vi "Periodic Tasks.vi"(8 "error in":errorcluster) -> ()   [LabVIEW 2017]
doc: "This VI runs in parallel to other tasks. It can contain as many user-defined periodic loops as you need. These can carry out PID or other sorts of timed response."
uses:
  <vilib>/Rock Robotics/WPI/Utilities/WPI_GetSetVariantRefNum.vi
  <vilib>/Rock Robotics/Network Tables/NT Write Numeric Array.vi
  <vilib>/Rock Robotics/Network Tables/NT Write Number.vi
  <vilib>/Rock Robotics/WPI/ThirdParty/Phoenix-LabVIEW/Motor Controller/Get/CTRE_Phoenix_MotorController_GetQuadratureData.vi
  <vilib>/Rock Robotics/WPI/ThirdParty/Phoenix-LabVIEW/Motor Controller/Get/CTRE_Phoenix_MotorController_GetOutputCurrent_Enhanced.vi
  <vilib>/Rock Robotics/WPI/ThirdParty/Phoenix-LabVIEW/Motor Controller/Get/CTRE_Phoenix_MotorController_GetVoltage.vi
  <vilib>/Rock Robotics/WPI/ThirdParty/Phoenix-LabVIEW/Motor Controller/Get/CTRE_Phoenix_MotorController_GetTemperature.vi
  <vilib>/Rock Robotics/Network Tables/NT Write Variant.vi
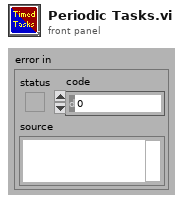
[diagram p1: front panel]
types:
  T1 = typedef "WPI_JoystickDevRef.ctl" = cluster{"Device":T2}
  T2 = typedef "WPI_JoystickDeviceEnum.ctl" = enum16{"USB 0", "USB 1", "USB 2", "USB 3", "USB 4", "USB 5"}
  T3 = typedef "WPI_AccelerometerDevRef.ctl" = cluster{"DevStatus":errorcluster, "Scaling":T4, "Analog Channels":T5, "I2C Bus":T7, "SPI Bus":T8, "Accel Range":T9, "ADXL Axes":T10, "Handle":i32, "Device Address":u8, "Accel Type":enum16{"Analog", "ADXL345 I2C", "ADXL345 SPI", "Internal", "ADXL362 SPI"}}
  T4 = typedef "WPI_AccelerometerScaling.ctl" = cluster{"Gain (VoltsPerG)":dbl, "Center Voltage":dbl}
  T5 = typedef "WPI_AccelerometerAnalogChannels.ctl" = cluster{"X-Axis":T6, "Y-Axis":T6, "Z-Axis":T6}
  T6 = typedef "FPGA_AIChannel.ctl" = enum8{"AI 0", "AI 1", "AI 2", "AI 3", "AI MXP 0", "AI MXP 1", "AI MXP 2", "AI MXP 3", "Invalid"}
  T7 = typedef "i2c_bus.ctl" = enum16{"I2C On-Board", "I2C MXP", "Invalid"}
  T8 = typedef "spi_bus.ctl" = enum16{"SPI On-Board, CS0", "SPI On-Board, CS1", "SPI On-Board, CS2", "SPI On-Board, CS3", "SPI MXP", "Invalid"}
  T9 = typedef "ADXL345 Range.ctl" = u8
  T10 = typedef "WPI_AccelerometerADXL345 Axes.ctl" = cluster{"X-Axis":bool, "Y-Axis":bool, "Z-Axis":bool}
  T11 = cluster{"X-Axis":dbl, "Y-Axis":dbl, "Z-Axis":dbl}
  T12 = typedef "WPI_GyroDevRef.ctl" = cluster{"DevStatus":errorcluster, "Analog Channel":T6, "Gain (VoltsPerDegree/Second)":dbl, "Gyro Type":enum16{"Analog", "XRS450"}, "Handle":i32, "SPI Bus":T8, "Device Found":bool, "Sample Rate":dbl, "Calibrate On Open":bool, "Offset":dbl}
  T13 = typedef "WPI_MotorControlDeviceRef.ctl" = cluster{"DeviceStatus":errorcluster, "Type":T14, "PWM":cluster{"PWM Channel":T15, "DeadBand":T16}, "CAN":cluster{"Device Number":u8, "SetOutput VI Ref":variant, "GetOutput VI Ref":variant, "Enable VI Ref":variant, "Disable VI Ref":variant, "Data":variant}, "Invert":bool, "DIO PWM":cluster{"PWM \"Enable\" Channel":T15, "DIOChannel":T17, "PWM Rate":dbl}}
  T14 = typedef "WPI_MotorControlType.ctl" = enum16{"PWM", "CAN", "DIO PWM"}
  T15 = typedef "FPGA_DIOPWMChannel.ctl" = enum8{"PWM 0", "PWM 1", "PWM 2", "PWM 3", "PWM 4", "PWM 5", "PWM 6", "PWM 7", "PWM 8", "PWM 9", "PWM MXP 0", "PWM MXP 1", "PWM MXP 2", "PWM MXP 3", "PWM MXP 4", "PWM MXP 5", "PWM MXP 6", "PWM MXP 7", "PWM MXP 8", "PWM MXP 9", "Invalid"}
  T16 = typedef "WPI_PWMDeadband.ctl" = cluster{"Name":string, "maxPositivePwm":i32, "minPositivePwm":i32, "centerPwm":i32, "maxNegativePwm":i32, "minNegativePwm":i32, "angularRange":u16}
  T17 = typedef "FPGA_DIOChannel.ctl" = enum8{"DIO 0", "DIO 1", "DIO 2", "DIO 3", "DIO 4", "DIO 5", "DIO 6", "DIO 7", "DIO 8", "DIO 9", "DIO MXP 0", "DIO MXP 1", "DIO MXP 2", "DIO MXP 3", "DIO MXP 4", "DIO MXP 5", "DIO MXP 6", "DIO MXP 7", "DIO MXP 8", "DIO MXP 9", "DIO MXP 10", "DIO MXP 11", "DIO MXP 12", "DIO MXP 13", "DIO MXP 14", "DIO MXP 15", "SPI Port CS1", "SPI Port CS2", "SPI Port CS3", "SPI Port MISO", "SPI Port MOSI", "Invalid"}
  T18 = cluster{"Temperature (C)":dbl, "Percent Output":dbl, "Output Voltage":dbl, "Bus Voltage":dbl, "Output Current":dbl}
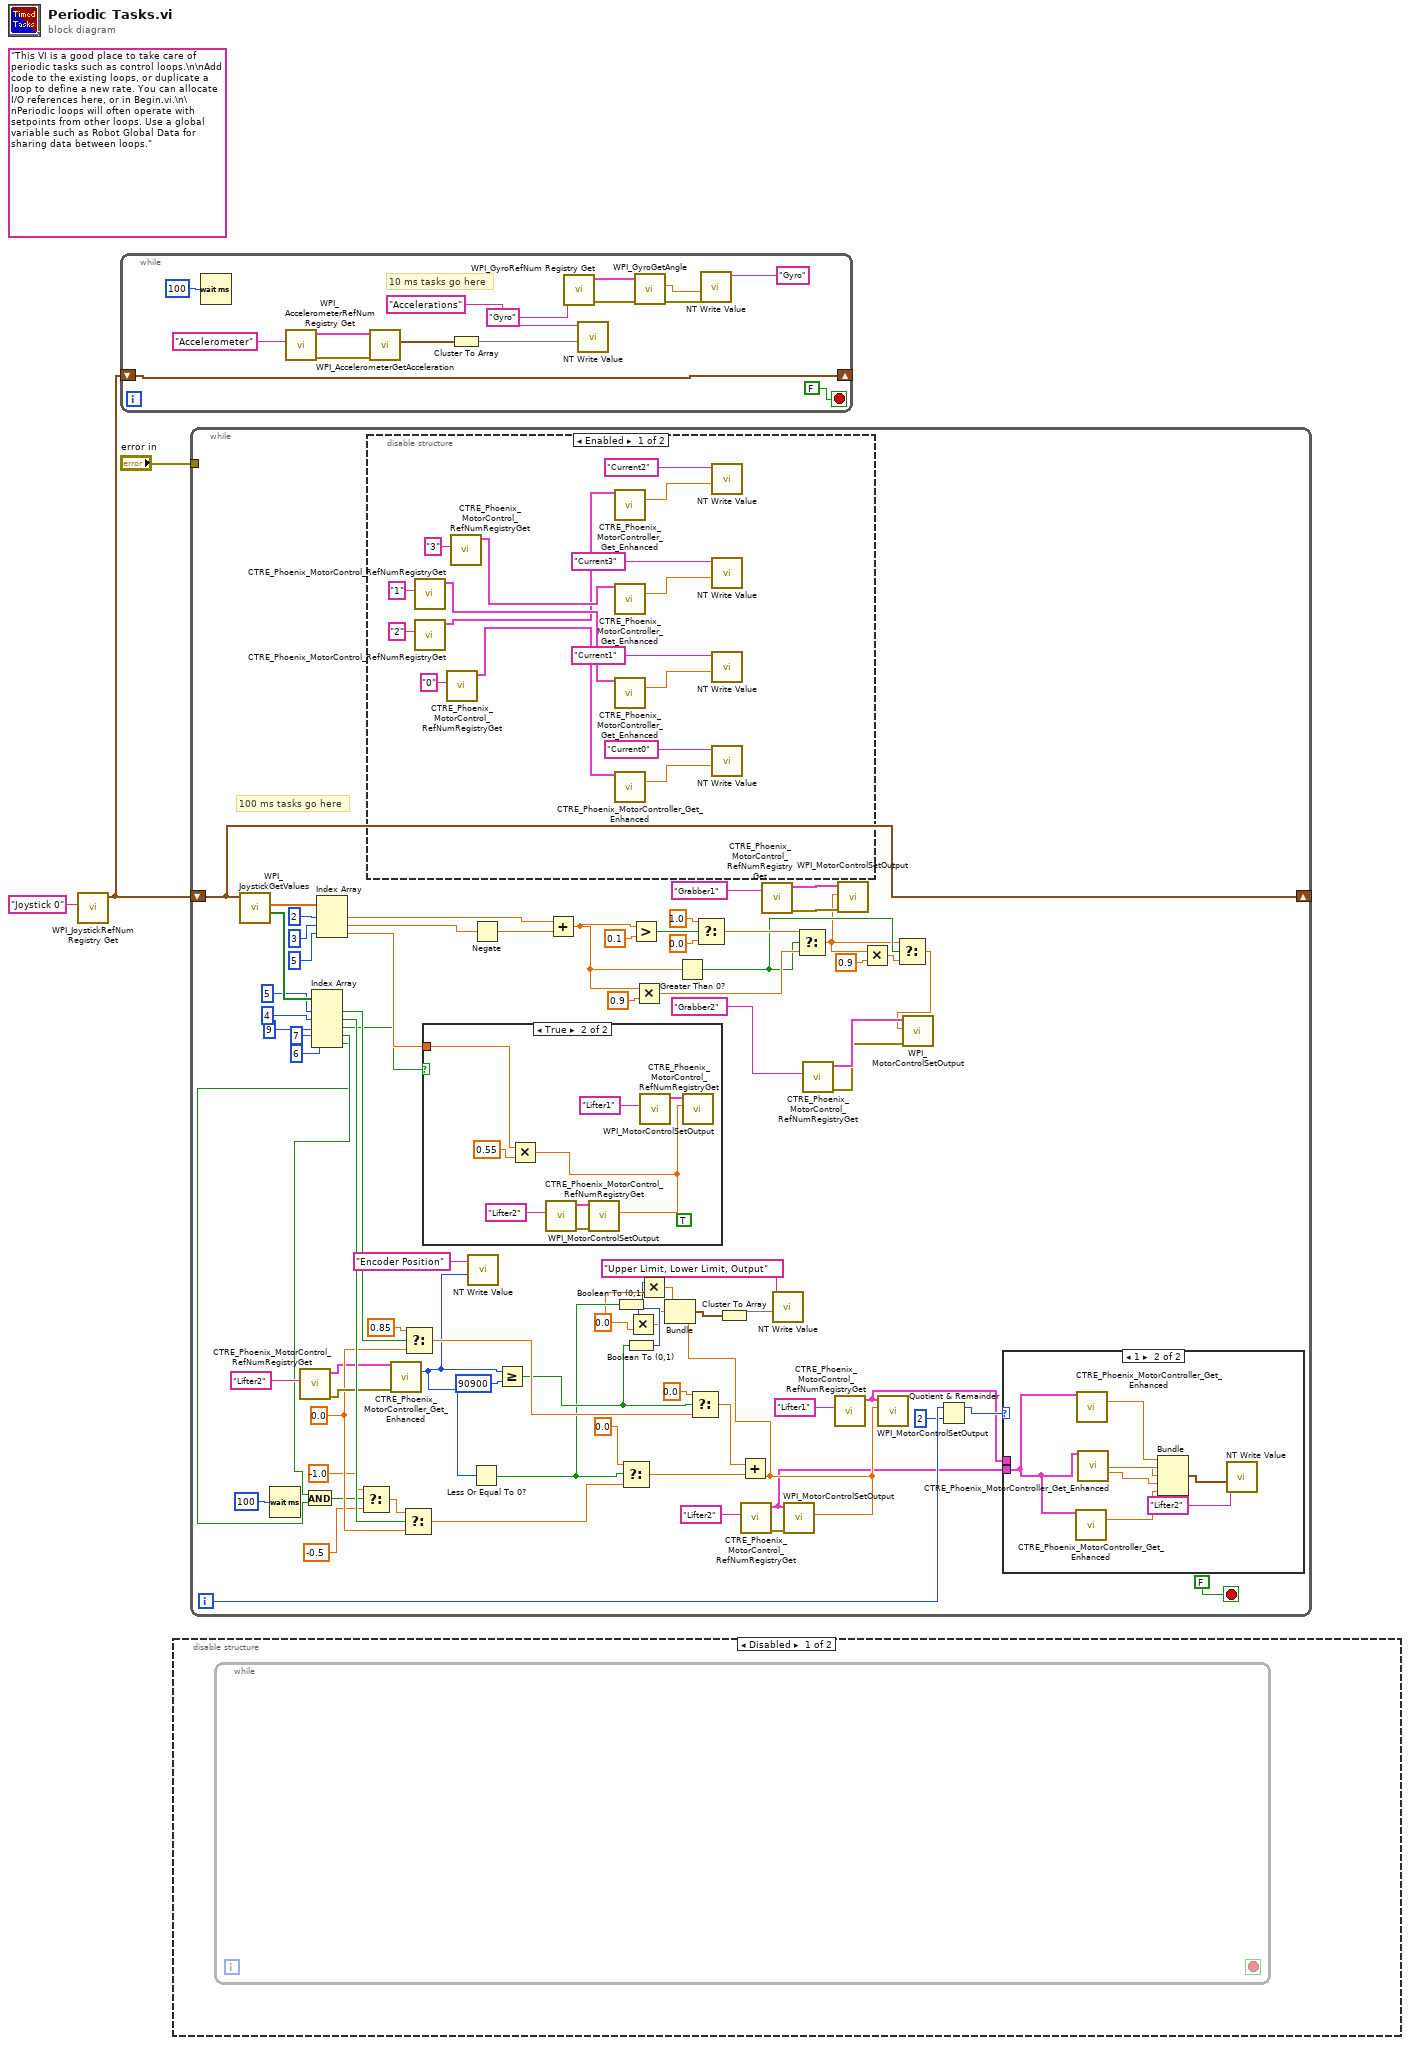
[diagram p0: block diagram]
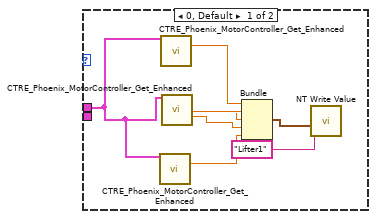
[diagram p3: hidden frame]
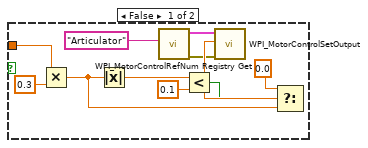
[diagram p5: hidden frame]
diagram:
  (unwired) "This VI is a good place to take care of periodic tasks such as control loops.\n\nAdd code to the existing loops, or duplicate a loop to define a new rate. You can allocate I/O references here, or in Begin.vi.\n\nPeriodic loops will often operate with setpoints from other loops. Use a global variable such as Robot Global Data for sharing data between loops."
  n1 = call <vilib>:"WPI_JoystickRefNum Registry Get.vi"("refnum name"="Joystick 0") -> ("JoystickDevRef"=w2:T1)  [unwired: 1 in, 9 out]
  n2 = while {
    shift-right: [w10] -> _
    shift-left: w2 -> [w10]
    stop <- FALSE stop-if-true
    # "10 ms tasks go here"
    n3 = Wait (ms)(milliseconds to wait=u32 100) -> ()  [unwired: 1 out]
    n4 = call <vilib>:"WPI_AccelerometerRefNum Registry Get.vi"("refnum name"="Accelerometer") -> ("error out"=w15:errorcluster, "AccelerometerDevRef"=w16:T3)  [unwired: 9 in]
    n5 = call <vilib>:"WPI_AccelerometerGetAcceleration.vi"("error in"=w15, "AccelerometerDevRef"=w16) -> ("Accelerations"=w12:T11)  [unwired: 7 in, 2 out]
    n6 = Cluster To Array(cluster=w12) -> (array=w11:dbl[])
    n7 = call <vilib>:"WPI_GyroRefNum Registry Get.vi"("refnum name"="Gyro") -> ("error out"=w8:errorcluster, "GyroDevRef"=w9:T12)  [unwired: 9 in]
    n8 = call-poly <vilib>:"NT Write Value.vi"("Numeric Array"=w11, "Name"="Accelerations") -> ()  [unwired: 9 in, 1 out]
    n9 = call <vilib>:"WPI_GyroGetAngle.vi"("error in"=w8, "GyroDevRef"=w9) -> ("error out"=w6:errorcluster, "Angle"=w7:dbl)  [unwired: 5 in, 3 out]
    n10 = call-poly <vilib>:"NT Write Value.vi"("error in"=w6, "Numeric"=w7, "Name"="Gyro") -> ()  [unwired: 8 in, 1 out]
  }
  n11 = disable-structure shown="Disabled" {
    frame Disabled {
      n12 = while {
        stop <- _ stop-if-true
      }
    }
    frame Enabled {
    }
  }
  n13 = while {
    shift-right: [w94] -> _
    shift-left: w2 -> [w94]
    tunnel: "error in" -> [_]
    i -> [w23]
    stop <- FALSE stop-if-true
    w46 = 0.0 ("y")
    w72 = 0.0 ("f")
    # "100 ms tasks go here"
    n14 = call <vilib>:"WPI_JoystickGetValues.vi"("JoystickDevRef"=w94) -> ("Buttons"=w93:bool[], "Axes"=w85:dbl[])  [unwired: 6 in, 3 out]
    n15 = Wait (ms)(milliseconds to wait=u32 100) -> ()  [unwired: 1 out]
    n16 = call <vilib>:"CTRE_Phoenix_MotorControl_RefNumRegistryGet.vi"("refnum name"="Lifter2") -> ("error out"=w87:errorcluster, "PhoenixMotorControlDevRef"=w68:T13)  [unwired: 9 in]
    n17 = Index Array(array=w93, index #1=5 ("index"), index #2=4 ("index"), index #3=9 ("index"), index #4=7 ("index"), index #5=6 ("index")) -> (element #1=w90:bool, element #2=w89:bool, element #3=w33:bool, element #4=w26:bool, element #5=w25:bool)
    n18 = And(x=w26, y=w25) -> (x .and. y?=w27:bool)
    n19 = Index Array(array=w85, index #1=2 ("index"), index #2=3 ("index"), index #3=5 ("index")) -> (element #1=w82:dbl, element #2=w75:dbl, element #3=w34:dbl)
    n20 = Select(t=-1.0, s=w27, f=-0.5) -> (s? t:f=w30:dbl)
    n21 = disable-structure shown="Enabled" {
      frame Enabled {
        n22 = call <vilib>:"CTRE_Phoenix_MotorControl_RefNumRegistryGet.vi"("refnum name"="1") -> ("PhoenixMotorControlDevRef"=w119:T13)  [unwired: 9 in, 1 out]
        n23 = call <vilib>:"CTRE_Phoenix_MotorControl_RefNumRegistryGet.vi"("refnum name"="2") -> ("PhoenixMotorControlDevRef"=w118:T13)  [unwired: 9 in, 1 out]
        n24 = call <vilib>:"CTRE_Phoenix_MotorControl_RefNumRegistryGet.vi"("refnum name"="0") -> ("PhoenixMotorControlDevRef"=w117:T13)  [unwired: 9 in, 1 out]
        n25 = call <vilib>:"CTRE_Phoenix_MotorControl_RefNumRegistryGet.vi"("refnum name"="3") -> ("PhoenixMotorControlDevRef"=w120:T13)  [unwired: 9 in, 1 out]
        n26 = call-poly <vilib>:"CTRE_Phoenix_MotorController_Get_Enhanced.vi"("PhoenixMotorControlDevRef"=w118) -> ("Output Current"=w126:dbl)  [unwired: 12 in, 2 out]
        n27 = call-poly <vilib>:"CTRE_Phoenix_MotorController_Get_Enhanced.vi"("PhoenixMotorControlDevRef"=w120) -> ("Output Current"=w125:dbl)  [unwired: 12 in, 2 out]
        n28 = call-poly <vilib>:"CTRE_Phoenix_MotorController_Get_Enhanced.vi"("PhoenixMotorControlDevRef"=w119) -> ("Output Current"=w127:dbl)  [unwired: 12 in, 2 out]
        n29 = call-poly <vilib>:"CTRE_Phoenix_MotorController_Get_Enhanced.vi"("PhoenixMotorControlDevRef"=w117) -> ("Output Current"=w128:dbl)  [unwired: 12 in, 2 out]
        n30 = call-poly <vilib>:"NT Write Value.vi"("Numeric"=w126, "Name"="Current2") -> ()  [unwired: 9 in, 1 out]
        n31 = call-poly <vilib>:"NT Write Value.vi"("Numeric"=w125, "Name"="Current3") -> ()  [unwired: 9 in, 1 out]
        n32 = call-poly <vilib>:"NT Write Value.vi"("Numeric"=w127, "Name"="Current1") -> ()  [unwired: 9 in, 1 out]
        n33 = call-poly <vilib>:"NT Write Value.vi"("Numeric"=w128, "Name"="Current0") -> ()  [unwired: 9 in, 1 out]
      }
      frame Disabled {
      }
    }
    n34 = call-poly <vilib>:"CTRE_Phoenix_MotorController_Get_Enhanced.vi"("PhoenixMotorControlDevRef"=w68, "error in"=w87) -> ("Quadrature Position"=w52:i32)  [unwired: 10 in, 3 out]
    n35 = Select(t=w30, s=w89, f=w72) -> (s? t:f=w59:dbl)
    n36 = Select(t=0.85, s=w90, f=w72) -> (s? t:f=w60:dbl)
    n37 = case shown="True" w33 {
      tunnel: w34 -> [w130 w140]
      frame False {
        n38 = Multiply(x=w130, y=0.3) -> (x*y=w138:dbl)
        n39 = Absolute Value(x=w138) -> (abs(x)=w137:dbl)
        n40 = call <vilib>:"WPI_MotorControlRefNum Registry Get.vi"("refnum name"="Articulator") -> ("error out"=w135:errorcluster, "MotorControlDevRef"=w134:T13)  [unwired: 9 in]
        n41 = Less?(x=w137, y=0.1) -> (x < y?=w136:bool)
        n42 = Select(t=0.0, s=w136, f=w138) -> (s? t:f=w139:dbl)
        n43 = call <vilib>:"WPI_MotorControlSetOutput.vi"("error in (no error)"=w135, "Output"=w139, "MotorControlDevRef"=w134) -> ()  [unwired: 6 in, 3 out]
      }
      frame True {
        (unwired) TRUE
        n44 = Multiply(x=w140, y=0.55) -> (x*y=w142:dbl)
        n45 = call <vilib>:"CTRE_Phoenix_MotorControl_RefNumRegistryGet.vi"("refnum name"="Lifter2") -> ("error out"=w143:errorcluster, "PhoenixMotorControlDevRef"=w146:T13)  [unwired: 9 in]
        n46 = call <vilib>:"WPI_MotorControlSetOutput.vi"("error in (no error)"=w143, "Output"=w142, "MotorControlDevRef"=w146) -> ()  [unwired: 6 in, 3 out]
        n47 = call <vilib>:"CTRE_Phoenix_MotorControl_RefNumRegistryGet.vi"("refnum name"="Lifter1") -> ("PhoenixMotorControlDevRef"=w144:T13)  [unwired: 9 in, 1 out]
        n48 = call <vilib>:"WPI_MotorControlSetOutput.vi"("Output"=w142, "MotorControlDevRef"=w144) -> ()  [unwired: 7 in, 3 out]
      }
    }
    n49 = call-poly <vilib>:"NT Write Value.vi"("Numeric"=w52, "Name"="Encoder Position") -> ()  [unwired: 9 in, 1 out]
    n50 = Less Or Equal To 0?(x=w52) -> (x <= 0?=w48:bool)
    n51 = Negate(x=w75) -> (-x=w74:dbl)
    n52 = Greater Or Equal?(x=w52, y=90900) -> (x >= y?=w49:bool)
    n53 = Add(x=w82, y=w74) -> (x+y=w63:dbl)
    n54 = Boolean To (0,1)(Boolean=w48) -> (0, 1=w43:i16)
    n55 = Select(t=0.0, s=w48, f=w59) -> (s? t:f=w55:dbl)
    n56 = Boolean To (0,1)(Boolean=w49) -> (0, 1=w45:i16)
    n57 = Multiply(x=w45, y=w46) -> (x*y=w44:dbl)
    n58 = Greater?(x=w63, y=0.1) -> (0:w61:bool)
    n59 = Multiply(x=w63, y=0.9) -> (x*y=w70:dbl)
    n60 = Multiply(x=w43, y=w46) -> (x*y=w42:dbl)
    n61 = Greater Than 0?(x=w63) -> (x > 0?=w40:bool)
    n62 = Select(t=0.0, s=w49, f=w60) -> (s? t:f=w56:dbl)
    n63 = Select(t=1.0 ("y"), s=w61, f=0.0) -> (s? t:f=w66:dbl)
    n64 = Add(x=w56, y=w55) -> (x+y=w51:dbl)
    n65 = Bundle(w42, w44, w51) -> (w41:cluster{dbl, dbl, dbl})  [unwired: 1 in]
    n66 = Cluster To Array(cluster=w41) -> (array=w47:dbl[])
    n67 = call <vilib>:"CTRE_Phoenix_MotorControl_RefNumRegistryGet.vi"("refnum name"="Lifter2") -> ("error out"=w53:errorcluster, "PhoenixMotorControlDevRef"=w21:T13)  [unwired: 9 in]
    n68 = call <vilib>:"CTRE_Phoenix_MotorControl_RefNumRegistryGet.vi"("refnum name"="Grabber1") -> ("error out"=w80:errorcluster, "PhoenixMotorControlDevRef"=w81:T13)  [unwired: 9 in]
    n69 = call-poly <vilib>:"NT Write Value.vi"("Numeric Array"=w47, "Name"="Upper Limit, Lower Limit, Output") -> ()  [unwired: 9 in, 1 out]
    n70 = call <vilib>:"WPI_MotorControlSetOutput.vi"("error in (no error)"=w53, "Output"=w51, "MotorControlDevRef"=w21) -> ()  [unwired: 6 in, 3 out]
    n71 = Select(t=w66, s=w40, f=w70) -> (s? t:f=w38:dbl)
    n72 = call <vilib>:"CTRE_Phoenix_MotorControl_RefNumRegistryGet.vi"("refnum name"="Grabber2") -> ("error out"=w78:errorcluster, "PhoenixMotorControlDevRef"=w79:T13)  [unwired: 9 in]
    n73 = call <vilib>:"CTRE_Phoenix_MotorControl_RefNumRegistryGet.vi"("refnum name"="Lifter1") -> ("PhoenixMotorControlDevRef"=w19:T13)  [unwired: 9 in, 1 out]
    n74 = call <vilib>:"WPI_MotorControlSetOutput.vi"("error in (no error)"=w80, "Output"=w38, "MotorControlDevRef"=w81) -> ()  [unwired: 6 in, 3 out]
    n75 = Multiply(x=w38, y=0.9) -> (x*y=w39:dbl)
    n76 = call <vilib>:"WPI_MotorControlSetOutput.vi"("Output"=w51, "MotorControlDevRef"=w19) -> ()  [unwired: 7 in, 3 out]
    n77 = Select(t=w38, s=w40, f=w39) -> (s? t:f=w36:dbl)
    n78 = call <vilib>:"WPI_MotorControlSetOutput.vi"("error in (no error)"=w78, "Output"=w36, "MotorControlDevRef"=w79) -> ()  [unwired: 6 in, 3 out]
    n79 = Quotient & Remainder(x=w23, y=2) -> (x-y*floor(x/y)=w24:i32)  [unwired: 1 out]
    n80 = case shown="1" w24 {
      tunnel: w21 -> [_ w107]
      tunnel: w19 -> [w97 _]
      frame 0, Default {
        n81 = call-poly <vilib>:"CTRE_Phoenix_MotorController_Get_Enhanced.vi"("PhoenixMotorControlDevRef"=w97) -> ("Output Current"=w100:dbl)  [unwired: 12 in, 2 out]
        n82 = call-poly <vilib>:"CTRE_Phoenix_MotorController_Get_Enhanced.vi"("PhoenixMotorControlDevRef"=w97) -> ("Temperature (C)"=w104:dbl)  [unwired: 12 in, 2 out]
        n83 = call-poly <vilib>:"CTRE_Phoenix_MotorController_Get_Enhanced.vi"("PhoenixMotorControlDevRef"=w97) -> ("Percent Output"=w103:dbl, "Output Voltage"=w102:dbl, "Bus Voltage"=w101:dbl)  [unwired: 10 in, 2 out]
        n84 = Bundle("Temperature (C)"=w104, "Percent Output"=w103, "Output Voltage"=w102, "Bus Voltage"=w101, "Output Current"=w100) -> (w99:T18)  [unwired: 1 in]
        n85 = call-poly <vilib>:"NT Write Value.vi"("Variant"=w99, "Name"="Lifter1") -> ()  [unwired: 9 in, 1 out]
      }
      frame 1 {
        n86 = call-poly <vilib>:"CTRE_Phoenix_MotorController_Get_Enhanced.vi"("PhoenixMotorControlDevRef"=w107) -> ("Output Current"=w108:dbl)  [unwired: 12 in, 2 out]
        n87 = call-poly <vilib>:"CTRE_Phoenix_MotorController_Get_Enhanced.vi"("PhoenixMotorControlDevRef"=w107) -> ("Temperature (C)"=w112:dbl)  [unwired: 12 in, 2 out]
        n88 = call-poly <vilib>:"CTRE_Phoenix_MotorController_Get_Enhanced.vi"("PhoenixMotorControlDevRef"=w107) -> ("Percent Output"=w111:dbl, "Output Voltage"=w110:dbl, "Bus Voltage"=w109:dbl)  [unwired: 10 in, 2 out]
        n89 = Bundle("Temperature (C)"=w112, "Percent Output"=w111, "Output Voltage"=w110, "Bus Voltage"=w109, "Output Current"=w108) -> (w106:T18)  [unwired: 1 in]
        n90 = call-poly <vilib>:"NT Write Value.vi"("Variant"=w106, "Name"="Lifter2") -> ()  [unwired: 9 in, 1 out]
      }
    }
  }
